vi "Main.vi"(11 "Error in":errorcluster) -> (15 "Error out":errorcluster)   [LabVIEW 2020, in "Data Communication Receiver.lvlib"]
doc: "This VI is used as a receiver for transmitted data which will receive data from queue notifier or occurrence."
uses:
  Data Communication Receiver.lvlib
  Typedefs/Received Data.ctl
  Typedefs/Queue operations.ctl
  Typedefs/State and data.ctl
  Typedefs/Data Cluster.ctl
  Typedefs/User event Operations.ctl
  Transmitter/Typedefs/User_Event_Operation.ctl
  Transmitter/Classes/Communication/Communication.lvclass
  Typedefs/User Event Stop Data.ctl
  Transmitter/Data Communication Transmitter.lvlib
  Transmitter/Classes/Children/Intra-Application/Children/Without data/Without Data.lvclass
panel:
  out "Occurrence ?":bool
  in  "Stop":bool
  out "Received Data":T1
  in  "Receive":bool
  # "DATA RECEIVER"
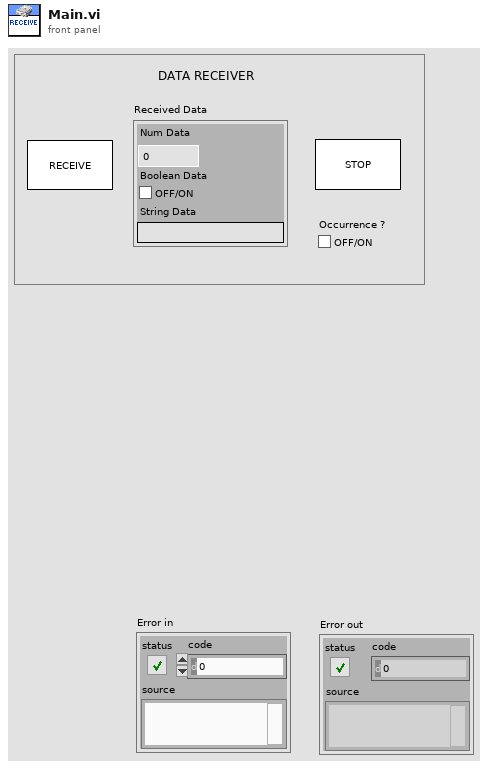
[diagram p1: front panel]
types:
  T1 = typedef "Data Communication Receiver.lvlib/Received Data.ctl" = cluster{"Num Data":dbl, "Boolean Data":bool, "String Data":string}
  T2 = typedef "Data Communication Transmitter.lvlib/User event Operations.ctl" = enum16{"Create", "Generate", "Get Ref", "destroy"}
  T3 = typedef "Data Communication Transmitter.lvlib/User_Event_Operation.ctl" = enum16{"Create", "Generate", "Destroy", "Get Ref"}
  T4 = typedef "Data Communication Receiver.lvlib/Data Cluster.ctl" = cluster{"Receive":bool, "Received Data":T1, "Occurrence ?":bool}
  T5 = typedef "Data Communication Receiver.lvlib/State and data.ctl" = cluster{"State":string, "Data":variant}
  T6 = typedef "Data Communication Receiver.lvlib/Queue operations.ctl" = enum16{"Create", "Enqueue", "Enstack", "Dequeue", "Flush", "Release"}
  T7 = typedef "Data Communication Receiver.lvlib/User Event Stop Data.ctl" = cluster{"Exit":bool}
  T8 = cluster{"Numeric data":dbl, "String data":string, "Boolean data":bool}
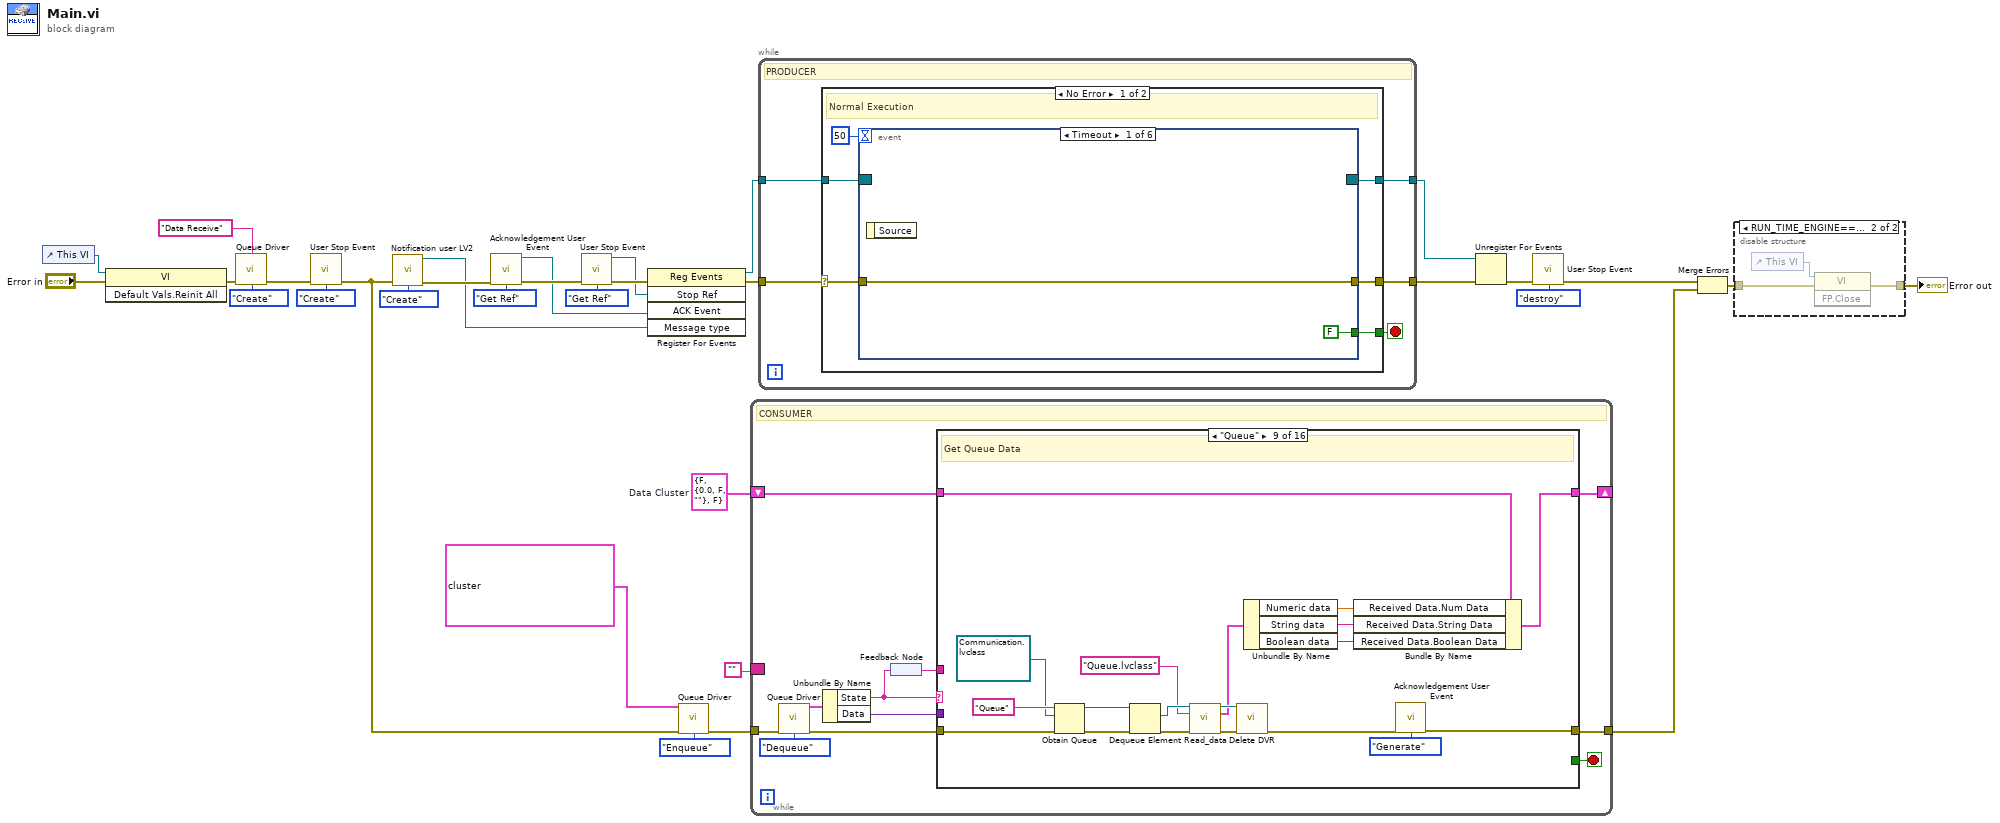
[diagram p0: block diagram]
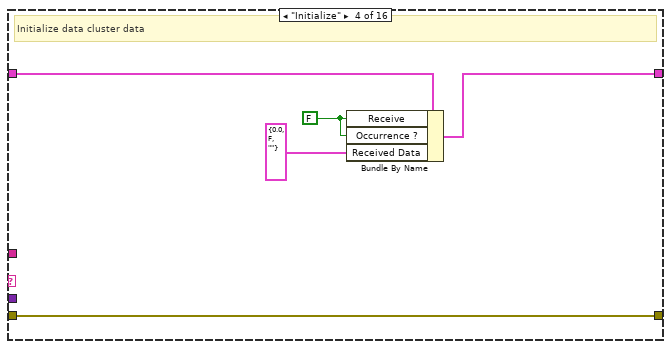
[diagram p6: hidden frame]
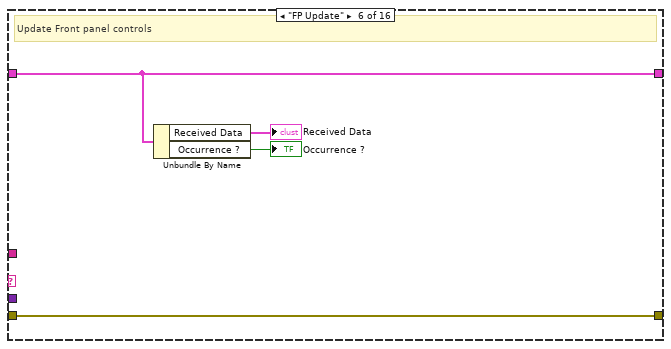
[diagram p8: hidden frame]
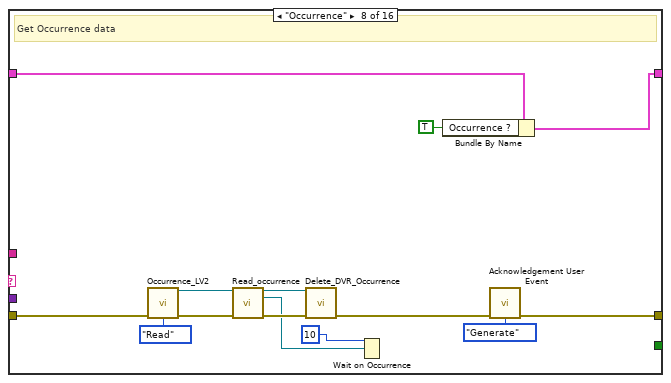
[diagram p10: hidden frame]
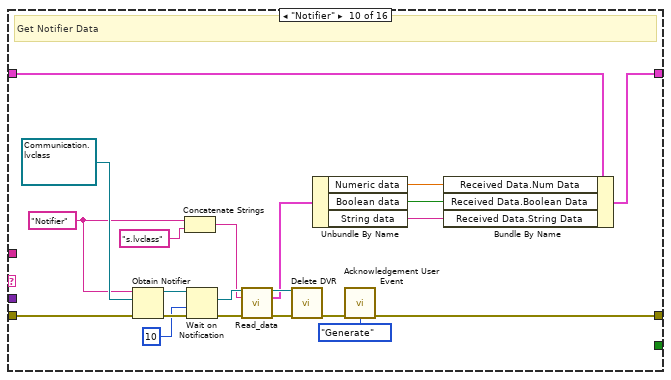
[diagram p11: hidden frame]
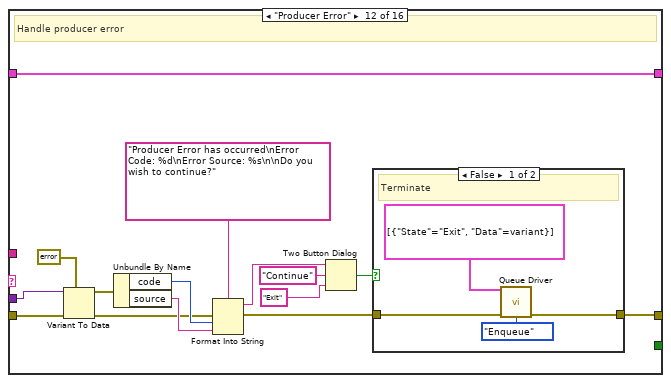
[diagram p13: hidden frame]
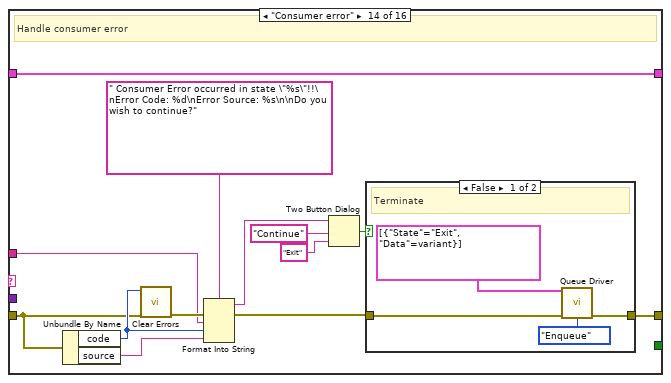
[diagram p16: hidden frame]
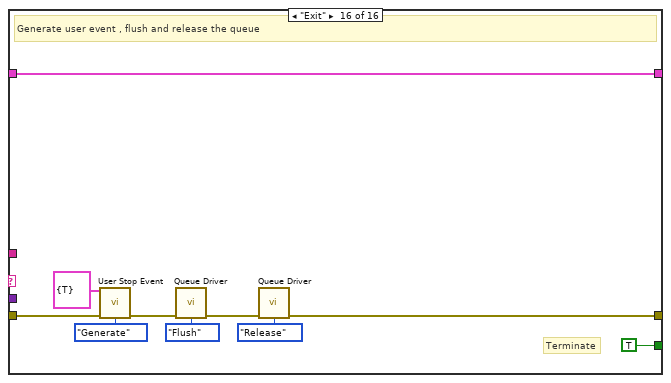
[diagram p19: hidden frame]
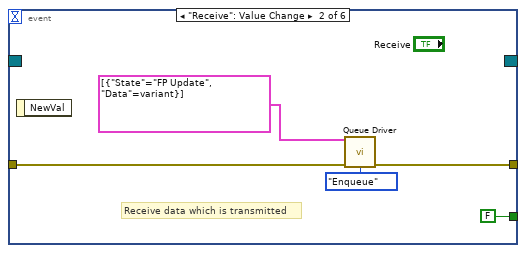
[diagram p20: hidden frame]
diagram:
  w16 = T4 {"Receive"=FALSE, "Received Data"={"Num Data"=0.0, "Boolean Data"=FALSE, "String Data"=""}, "Occurrence ?"=FALSE}  # Data Cluster
  n1 = control-ref of="This VI"() -> (w29:refnum<vi>)
  n2 = invoke class="VI" method="Default Vals.Reinit All"(reference=w29, error in="Error in") -> (error out=w28:errorcluster)  [unwired: 1 in, 2 out]
  n3 = call "Queue Driver.vi"("Name"="Data Receive", "Error in"=w28, "Operations"=Queue_operations."Create") -> ("Error out"=w2:errorcluster)  [unwired: 11 in, 1 out]
  n4 = call "User Stop Event.vi"("Error in"=w2, "Operations"=User_event_Operations."Create") -> ("Error out"=w1:errorcluster)  [unwired: 12 in, 1 out]
  n5 = call "Notification user LV2.vi"("Error In"=w1, "Operation"=User_Event_Operation."Create") -> ("Message type"=w6:refnum<user-event>, "Error Out"=w7:errorcluster)  [unwired: 12 in]
  n6 = call "Acknowledgement User Event.vi"("Error in"=w7, "Operations"=User_event_Operations."Get Ref") -> ("ACK Event"=w11:refnum<user-event>, "Error out"=w13:errorcluster)  [unwired: 12 in]
  n7 = call "User Stop Event.vi"("Error in"=w13, "Operations"=User_event_Operations."Get Ref") -> ("Stop Ref"=w17:refnum<user-event>, "Error out"=w20:errorcluster)  [unwired: 12 in]
  n8 = register-events(error in=w20, w17, w11, w6) -> (reference out=w18:refnum<event-registration>, error out=w19:errorcluster)  [unwired: 1 in]
  n9 = call "Queue Driver.vi"("Enqueue Elements"=T5[] [{"State"="Initialize", "Data"=variant}, {"State"="FP Update", "Data"=variant}], "Error in"=w1, "Operations"=Queue_operations."Enqueue") -> ("Error out"=w23:errorcluster)  [unwired: 11 in, 1 out]
  n10 = while {
    border: "" -> [_]
    tunnel: w23 -> [w41]
    tunnel: [w43] -> w32
    shift-right: [w33] -> _
    shift-left: w16 -> [w34]
    stop <- w35 stop-if-true
    # "CONSUMER"
    n11 = call "Queue Driver.vi"("Error in"=w41, "Operations"=Queue_operations."Dequeue") -> ("Dequeued Element"=w39:T5, "Error out"=w40:errorcluster)  [unwired: 12 in]
    n12 = Unbundle By Name(w39) -> ("State"=w38:string, "Data"=w36:variant)
    n13 = feedback-in #1(w38) -> ()
    n14 = feedback #1() -> (w37:string)
    n15 = case shown="\"Queue\"" w38 {
      tunnel: w40 -> [w45 w47 w49 w54 w56 w60 w62 w75 w95 w116 w118 w126 w140 w146 w160 w163]
      tunnel: [w45 w47 w49 w54 w56 w60 w62 w63 w86 w109 w118 w120 w140 w142 w160 w167] -> w43
      tunnel: w37 -> [_ _ _ _ _ _ _ _ _ _ _ _ _ w145 _ _]
      tunnel: w36 -> [_ _ _ _ _ _ _ _ _ _ _ w125 _ _ _ _]
      tunnel: [_ _ _ _ _ _ _ _ _ _ _ _ _ _ _ TRUE] -> w35
      tunnel: w34 -> [w44 w46 w48 w53 w55 w59 w61 w69 w92 w112 w117 w119 w139 w141 w159 w161]
      tunnel: [w44 w46 w48 w52 w55 w59 w61 w68 w91 w111 w117 w119 w139 w141 w159 w161] -> w33
      frame "/***Application Related***/" {
      }
      frame "Poll", Default {
        # "Application Default handling"
      }
      frame "/***Initialize***/" {
      }
      frame "Initialize" {
        w51 = FALSE ("Receive")
        # "Initialize data cluster data"
        n16 = Bundle By Name(cluster=w53, "Receive"=w51, "Occurrence ?"=w51, "Received Data"=T1 {"Num Data"=0.0, "Boolean Data"=FALSE, "String Data"=""}) -> (w52:T4)
      }
      frame "/***FP Related***/" {
      }
      frame "FP Update" {
        # "Update Front panel controls"
        n17 = Unbundle By Name(w59) -> ("Received Data"=→"Received Data":T1, "Occurrence ?"=→"Occurrence ?":bool)
      }
      frame "/*** data received***/" {
      }
      frame "Occurrence" {
        # "Get Occurrence data"
        n18 = call "Occurrence_LV2.vi"("Error In"=w75, "Operation"=enum16{"Init", "Read", "Write"}."Read") -> ("Without data DVR reference out"=w71:refnum<data-value>, "Error Out"=w74:errorcluster)  [unwired: 12 in]
        n19 = call "Read_occurrence.vi"("Without data DVR reference in"=w71, "error in (no error)"=w74) -> ("Without data DVR reference out"=w70:refnum<data-value>, "Occurrence Ref"=w72:refnum<k4>, "error out"=w73:errorcluster)  [unwired: 11 in]
        n20 = call "Delete_DVR_Occurrence.vi"("Without data DVR reference"=w70, "error in (no error)"=w73) -> ("error out"=w64:errorcluster)  [unwired: 13 in]
        n21 = Wait on Occurrence(2:w72, 3:10 ("ms timeout (-1)")) -> ()  [unwired: 1 in, 1 out]
        n22 = Bundle By Name(cluster=w69, "Occurrence ?"=TRUE) -> (w68:T4)
        n23 = call "Acknowledgement User Event.vi"("Error in"=w64, "Operations"=User_event_Operations."Generate") -> ("Error out"=w63:errorcluster)  [unwired: 12 in, 1 out]
      }
      frame "Queue" {
        # "Get Queue Data"
        n24 = Obtain Queue(name (unnamed)="Queue", element data type=refnum<data-value> refnum ("DVR Out"), error in (no error)=w95) -> (queue out=w93:refnum<queue>, error out=w94:errorcluster)  [unwired: 2 in, 1 out]
        n25 = Dequeue Element(queue=w93, error in (no error)=w94) -> (element=w82:refnum<data-value>, error out=w85:errorcluster)  [unwired: 1 in, 2 out]
        n26 = call "Read_data.vi"("notification"=w82, "Type"="Queue.lvclass", "error in (no error)"=w85) -> ("notification out"=w81:refnum<data-value>, "DATA"=w80:T8, "error out"=w84:errorcluster)  [unwired: 10 in]
        n27 = call "Delete DVR.vi"("DVR In"=w81, "error in (no error)"=w84) -> ("error out"=w83:errorcluster)  [unwired: 13 in]
        n28 = Unbundle By Name(w80) -> ("Numeric data"=w90:dbl, "String data"=w89:string, "Boolean data"=w88:bool)
        n29 = Bundle By Name(cluster=w92, "Received Data.Num Data"=w90, "Received Data.String Data"=w89, "Received Data.Boolean Data"=w88) -> (w91:T4)
        n30 = call "Acknowledgement User Event.vi"("Error in"=w83, "Operations"=User_event_Operations."Generate") -> ("Error out"=w86:errorcluster)  [unwired: 12 in, 1 out]
      }
      frame "Notifier" {
        w98 = "Notifier" ("name (unnamed)")
        # "Get Notifier Data"
        n31 = Obtain Notifier(name (unnamed)=w98, notification data type=refnum<data-value> refnum ("DVR Out"), error in (no error)=w116) -> (notifier out=w114:refnum<notifier>, error out=w115:errorcluster)  [unwired: 1 in, 1 out]
        n32 = Concatenate Strings(w98, "s.lvclass" ("string")) -> (w97:string)
        n33 = Wait on Notification(notifier=w114, timeout in ms (-1)=10, error in (no error)=w115) -> (notification=w99:refnum<data-value>, error out=w107:errorcluster)  [unwired: 1 in, 2 out]
        n34 = call "Read_data.vi"("notification"=w99, "Type"=w97, "error in (no error)"=w107) -> ("notification out"=w106:refnum<data-value>, "DATA"=w104:T8, "error out"=w105:errorcluster)  [unwired: 10 in]
        n35 = call "Delete DVR.vi"("DVR In"=w106, "error in (no error)"=w105) -> ("error out"=w108:errorcluster)  [unwired: 13 in]
        n36 = Unbundle By Name(w104) -> ("Numeric data"=w103:dbl, "Boolean data"=w102:bool, "String data"=w101:string)
        n37 = call "Acknowledgement User Event.vi"("Error in"=w108, "Operations"=User_event_Operations."Generate") -> ("Error out"=w109:errorcluster)  [unwired: 12 in, 1 out]
        n38 = Bundle By Name(cluster=w112, "Received Data.Num Data"=w103, "Received Data.Boolean Data"=w102, "Received Data.String Data"=w101) -> (w111:T4)
      }
      frame "/***Producer Error***/" {
      }
      frame "Producer Error" {
        # "Handle producer error"
        n39 = Variant To Data(error in=w126, type=errorcluster {"status"=FALSE, "code"=0, "source"=""} ("Error out"), Variant=w125) -> (data=w124:errorcluster, error out=w123:errorcluster)
        n40 = Unbundle By Name(w124) -> ("code"=w132:i32, "source"=w131:string)
        n41 = Format Into String(format string="Producer Error has occurred\nError Code: %d\nError Source: %s\n\nDo you wish to continue?", error in=w123, w132, w131) -> (resulting string=w130:string, error out=w122:errorcluster)  [unwired: 1 in]
        n42 = Two Button Dialog(message=w130, 1:"Exit" ("F button name (\"Cancel\")"), 2:"Continue" ("T button name (\"OK\")")) -> (T button?=w121:bool)
        n43 = case shown="False" w121 {
          tunnel: w122 -> [w136 w138]
          tunnel: [w135 w138] -> w120
          frame False {
            # "Terminate"
            n44 = call "Queue Driver.vi"("Enqueue Elements"=T5[] [{"State"="Exit", "Data"=variant}], "Error in"=w136, "Operations"=Queue_operations."Enqueue") -> ("Error out"=w135:errorcluster)  [unwired: 11 in, 1 out]
          }
          frame True {
            # "Continue"
          }
        }
      }
      frame "/***Consumer Error***/" {
      }
      frame "Consumer error" {
        # "Handle consumer error"
        n45 = Unbundle By Name(w146) -> ("code"=w151:i32, "source"=w147:string)
        n46 = call <vilib>:"Clear Errors.vi"("error in (no error)"=w146, "specific error code to clear (0: all)"=w151) -> ("error out"=w153:errorcluster)  [unwired: 4 in, 1 out]
        n47 = Format Into String(format string=" Consumer Error occurred in state \"%s\"!!\nError Code: %d\nError Source: %s\n\nDo you wish to continue?", error in=w153, w145, w151, w147) -> (resulting string=w150:string, error out=w143:errorcluster)  [unwired: 1 in]
        n48 = Two Button Dialog(message=w150, 1:"Exit" ("F button name (\"Cancel\")"), 2:"Continue" ("T button name (\"OK\")")) -> (T button?=w144:bool)
        n49 = case shown="False" w144 {
          tunnel: w143 -> [w156 w158]
          tunnel: [w155 w158] -> w142
          frame False {
            # "Terminate"
            n50 = call "Queue Driver.vi"("Enqueue Elements"=T5[] [{"State"="Exit", "Data"=variant}], "Error in"=w156, "Operations"=Queue_operations."Enqueue") -> ("Error out"=w155:errorcluster)  [unwired: 11 in, 1 out]
          }
          frame True {
            # "Continue"
          }
        }
      }
      frame "/***Exit***/" {
      }
      frame "Exit" {
        # "Terminate"
        # "Generate user event , flush and release the queue"
        n51 = call "User Stop Event.vi"("Stop"=T7 {"Exit"=TRUE}, "Error in"=w163, "Operations"=User_event_Operations."Generate") -> ("Error out"=w164:errorcluster)  [unwired: 11 in, 1 out]
        n52 = call "Queue Driver.vi"("Error in"=w164, "Operations"=Queue_operations."Flush") -> ("Error out"=w166:errorcluster)  [unwired: 12 in, 1 out]
        n53 = call "Queue Driver.vi"("Error in"=w166, "Operations"=Queue_operations."Release") -> ("Error out"=w167:errorcluster)  [unwired: 12 in, 1 out]
      }
    }
  }
  n54 = while {
    tunnel: [w175] -> w10
    tunnel: w19 -> [w174]
    tunnel: w18 -> [w173]
    tunnel: [w171] -> w8
    stop <- w172 stop-if-true
    # "PRODUCER"
    n55 = case shown="No Error" w174 {
      selector: w174 -> [w179 w220]
      tunnel: [w180 w215] -> w175
      tunnel: w173 -> [w178 w210]
      tunnel: [w177 FALSE] -> w172
      tunnel: [w176 w210] -> w171
      frame No Error {
        # "Normal Execution"
        n56 = event shown="[0] Timeout" {
          selector: w178 -> [_ _ _ _ _ _]
          dyn-events: [_ _ _ _ _ _] -> w176
          timeout: 50 -> [_ _ _ _ _ _]
          tunnel: [w183 w185 w189 w195 w204 w209] -> w180
          tunnel: w179 -> [w183 w186 w190 w200 w205 w209]
          tunnel: [FALSE FALSE TRUE FALSE TRUE TRUE] -> w177
          event Timeout {
            n57 = event-data() -> ()  [unwired: 1 in, 1 out]
          }
          event "Receive": Value Change {
            # "Receive data which is transmitted"
            n58 = event-data() -> ()  [unwired: 1 in, 1 out]
            n59 = call "Queue Driver.vi"("Enqueue Elements"=T5[] [{"State"="FP Update", "Data"=variant}], "Error in"=w186, "Operations"=Queue_operations."Enqueue") -> ("Error out"=w185:errorcluster)  [unwired: 11 in, 1 out]
          }
          event "Stop": Value Change {
            n60 = event-data() -> ()  [unwired: 1 in, 1 out]
            n61 = call "Queue Driver.vi"("Enqueue Elements"=T5[] [{"State"="Exit", "Data"=variant}], "Error in"=w190, "Operations"=Queue_operations."Enqueue") -> ("Error out"=w189:errorcluster)  [unwired: 11 in, 1 out]
          }
          event User Event {
            # "Get Message type from transmitter"
            n62 = event-data() -> ("Message type"=w198:string)  [unwired: 1 in]
            n63 = Bundle By Name(cluster=T5 {"State"="", "Data"=variant} ("Dequeued Element"), "State"=w198) -> (w197:T5)
            n64 = Build Array(w197) -> (w196:T5[])
            n65 = call "Queue Driver.vi"("Enqueue Elements"=w196, "Error in"=w200, "Operations"=Queue_operations."Enqueue") -> ("Error out"=w195:errorcluster)  [unwired: 11 in, 1 out]
          }
          event Panel Close? {
            n66 = event-data() -> ()  [unwired: 1 in, 1 out]
            n67 = call "Queue Driver.vi"("Enqueue Elements"=T5[] [{"State"="Exit", "Data"=variant}], "Error in"=w205, "Operations"=Queue_operations."Enqueue") -> ("Error out"=w204:errorcluster)  [unwired: 11 in, 1 out]
            n68 = event-data("Discard?"=TRUE) -> ()  [unwired: 1 in, 1 out]
          }
          event User Event {
            n69 = event-data() -> ()  [unwired: 1 in, 1 out]
          }
        }
      }
      frame Error {
        # "Handle Producer Error"
        n70 = To Variant(anything=w220) -> (Variant=w218:variant)
        n71 = Bundle By Name(cluster=T5 {"State"="", "Data"=variant} ("Dequeued Element"), "State"="Producer Error", "Data"=w218) -> (w213:T5)
        n72 = call <vilib>:"Clear Errors.vi"("error in (no error)"=w220) -> ("error out"=w216:errorcluster)  [unwired: 5 in, 1 out]
        n73 = Build Array(w213) -> (w212:T5[])
        n74 = call "Queue Driver.vi"("Enqueue Elements"=w212, "Error in"=w216, "Operations"=Queue_operations."Enqueue") -> ("Error out"=w215:errorcluster)  [unwired: 11 in, 1 out]
      }
    }
  }
  n75 = Unregister For Events(event registration refnum=w8, error in=w10) -> (error out=w9:errorcluster)
  n76 = call "User Stop Event.vi"("Error in"=w9, "Operations"=User_event_Operations."destroy") -> ("Error out"=w14:errorcluster)  [unwired: 12 in, 1 out]
  n77 = Merge Errors(w14, w32) -> (w31:errorcluster)
  n78 = disable-structure shown="RUN_TIME_ENGINE==True" {
    disable-tunnel: w31 -> [w221 w223]
    disable-tunnel: [w221 w222] -> w30
    frame condition #0 (active) {
    }
    frame condition #1 {
      n79 = control-ref of="This VI"() -> (w224:refnum<vi>)
      n80 = invoke class="VI" method="FP.Close"(reference=w224, error in=w223) -> (error out=w222:errorcluster)  [unwired: 1 in, 2 out]
    }
  }
  "Error out" <- w30
